vi "ExSpectralCalMovCollect.vi"() -> ()   [LabVIEW 2010]
panel:
  out "XY Graph":T1(graph)
  in  "Pixel Width (microns)":dbl=25.0 format="%.2f"
  in  "Magnification":dbl=1.0 format="%.2f"
  in  "Detector Angle (degrees)":dbl=1.0 format="%.2f"
  in  "Inclusion Angle (degrees)":dbl=1.0 format="%.2f"
  in  "Focal Length (mm)":dbl=300.0 format="%.2f"
  in  "Slope Adjust":dbl format="%.2f"
  in  "Center Offset":dbl format="%.2f"
  out "Current Wavelength":string
  in  "Increment Wavelength":dbl=50.0 format="%.2f"
  in  "End Wavelength":dbl=700.0 format="%.2f"
  in  "Start Wavelength":dbl format="%.2f"
  in  "Grating Speed":dbl=2000.0 min=1.0 step=1.0 format="%.2f"
  in  "Grating number":i16=1 min=1 max=100 step=1
  in  "Temperature":dbl=-10.0 format="%.2f"
  in  "Exposure":dbl min=0.0 step=0.001 format="%.3f"
  in  "stop":bool
  out "error out":errorcluster
  in  "error in (no error)":errorcluster
  # "ExSpectralCalMovCollect.vi\n(Normal Spectrograph via\nUSB/COM port)\nNote that appropriate calibration\ninformation for the spectrometer\nmust be entered before running.Camera and Spectrometer control.  This vi will open both the camera and spectrograph.  It will then move the grating to the Start Wavelength.  Data will then be collected and displayed.  The sequence will be repeated after moving the grating by the Increment Wavelength until the End Wavelength is reached.  At that time, data collection will continue until the STOP button is hit. The display will\nshow an updated calibration in nm."
  # "NOTES:\nIf required, a properly configured camera .ini file must be present for camera operation.\n\nThe properly configured spectrometer .ini file must be present in the LabVIEW folder for spectrograph operation.\n\nConsult the documentation for more information on how to configure these files."
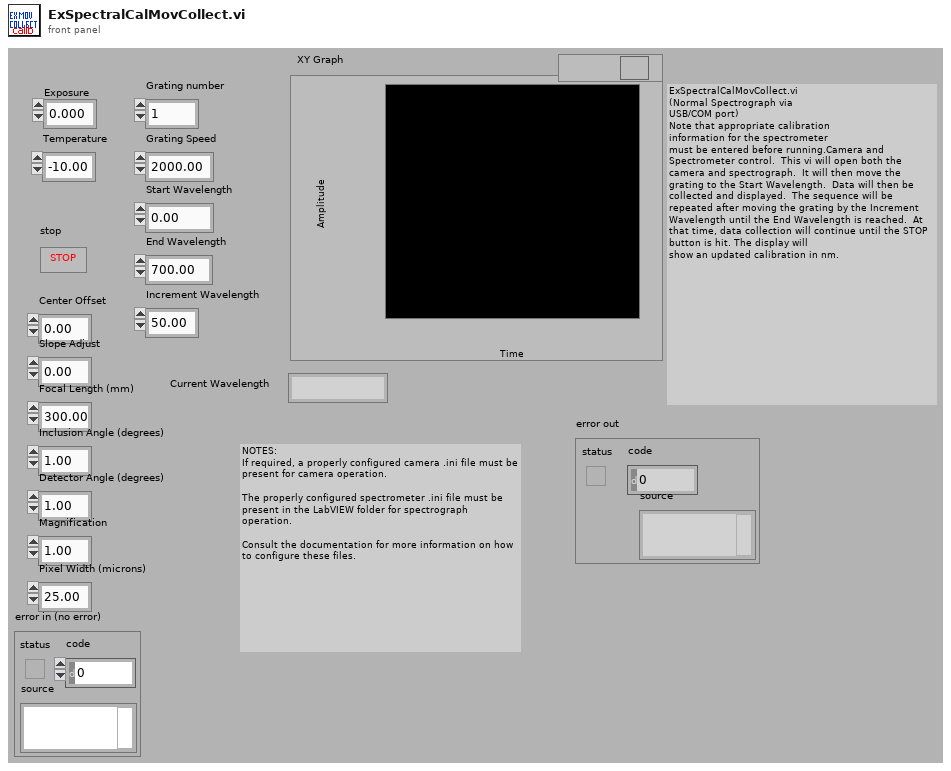
[diagram p1: front panel]
types:
  T1 = cluster{"Calibrated Array":dbl[], "Array F32":sgl[]}
  T2 = cluster{"Center Offset":dbl, "Slope Adjust":dbl, "Focal Length (mm)":dbl, "Inclusion Angle (degrees)":dbl, "Detector Angle (degrees)":dbl, "Magnification":dbl, "Pixel Width (microns)":dbl}
  T3 = cluster{"Camera Handle":u32, "Pulser Handle":u32, "File Handle":u32, "Display Handle":u32, "Image Handle":u32}
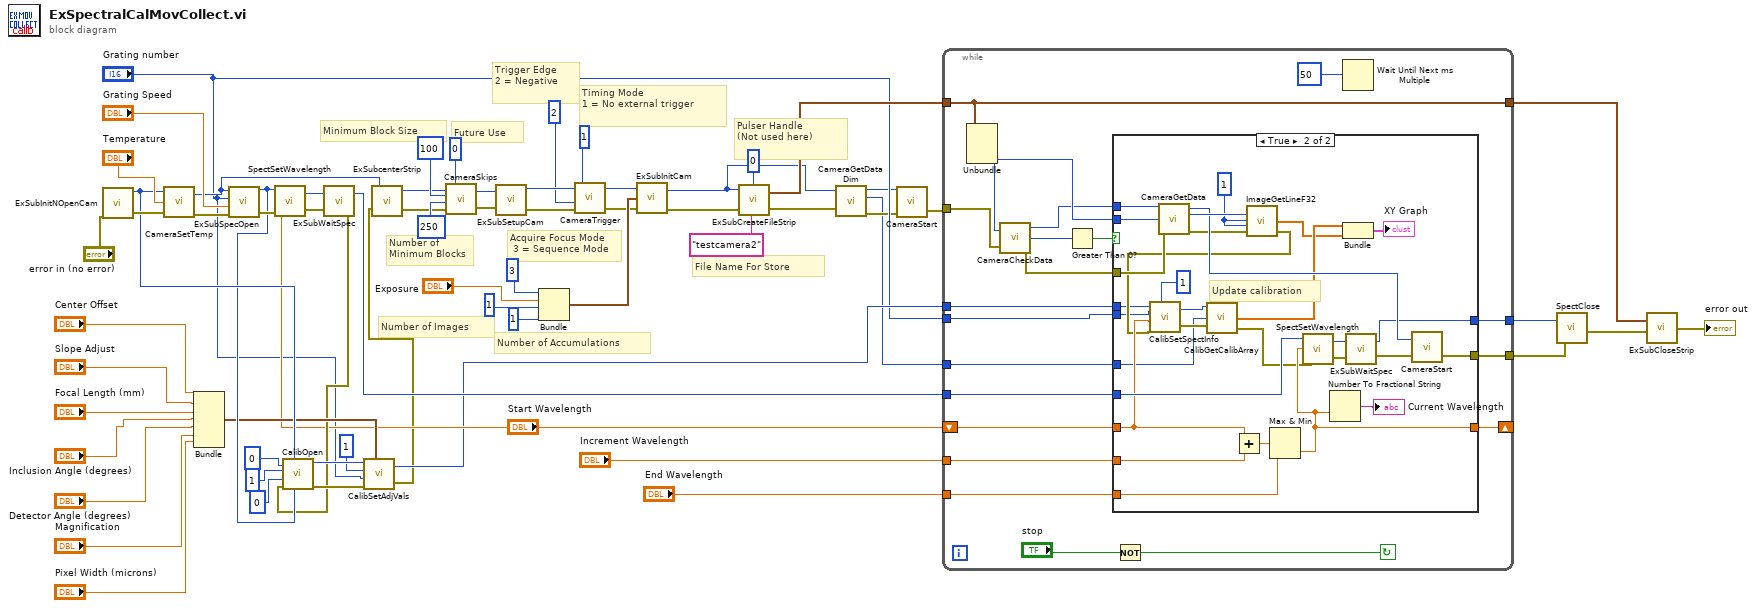
[diagram p0: block diagram]
diagram:
  # "Pulser Handle\n(Not used here)"
  # "Trigger Edge\n2 = Negative"
  # "Timing Mode\n1 = No external trigger"
  # "Future Use"
  # "Number of Minimum Blocks"
  # "Minimum Block Size"
  # "Number of Images"
  # "Number of Accumulations"
  # "Acquire Focus Mode\n 3 = Sequence Mode"
  # "File Name For Store"
  n1 = call "ExSubInitNOpenCam.vi"("error in (no error)"="error in (no error)") -> ("Camera Handle"=w25:u32, "error out"=w29:errorcluster)
  n2 = call <userlib>:"CameraSetTemp.vi"("error in (no error)"=w29, "Temperature"="Temperature", "Camera Handle"=w25) -> ("error out"=w30:errorcluster, "Camera Handle"=w22:u32)
  n3 = Bundle("Center Offset"="Center Offset", "Slope Adjust"="Slope Adjust", "Focal Length (mm)"="Focal Length (mm)", "Inclusion Angle (degrees)"="Inclusion Angle (degrees)", "Detector Angle (degrees)"="Detector Angle (degrees)", "Magnification"="Magnification", "Pixel Width (microns)"="Pixel Width (microns)") -> (w14:T2)  [unwired: 1 in]
  n4 = call "ExSubSpecOpen.vi"("error in (no error)"=w30, "Grating speed"="Grating Speed", "Grating number"="Grating number", "Camera Handles"=w22) -> ("error out"=w35:errorcluster, "Spectrometer Handle"=w23:u32)  [unwired: 1 out]
  n5 = call <userlib>:"SpectSetWavelength.vi"("error in"=w35, "Wavelength"="Start Wavelength", "Spectrometer Handle"=w23) -> ("error out"=w39:errorcluster, "Spectrumeter Handle"=w38:u32)
  n6 = call "ExSubWaitSpec.vi"("error in (no error)"=w39, "Spectrometer Handle"=w38) -> ("error out"=w10:errorcluster, "Spectrometer handle"=w37:u32)
  n7 = call <userlib>:"CalibOpen.vi"("Spectrometer Handle"=w23, "Detector Handle"=w25, "error in"=w10, "Detector Position"=0, "Calibration Type"=1, "Calibration Device ID"=0) -> ("error out"=w12:errorcluster, "Calibration Handle"=w13:u32)
  n8 = call <userlib>:"CalibSetAdjVals.vi"("Calibration Handle"=w13, "Turret Number"=1, "Grating Number"="Grating number", "error in"=w12, "Spectrometer Calibration Parameters"=w14) -> ("Calibration Handle"=w8:u32, "error out"=w6:errorcluster)
  n9 = call "ExSubcenterStrip.vi"("error in (no error)"=w6, "Camera Handle"=w22) -> ("error out"=w41:errorcluster, "Camera Handle"=w42:u32)
  n10 = call <userlib>:"CameraSkips.vi"("Camera Handle"=w42, "Minimum Block Size"=100, "Number of Minimum blocks"=250, "error in"=w41, "Type of Skips"=0) -> ("Camera Handle"=w44:u32, "error out"=w43:errorcluster)
  n11 = call "ExSubSetupCam.vi"("error in (no error)"=w43, "Camera Handle"=w44) -> ("error out"=w49:errorcluster, "Camera Handle"=w53:u32)
  n12 = Bundle(3, "Exposure"="Exposure", 1, 1) -> (w60:cluster{i32, "Exposure":dbl, i32, i32})  [unwired: 1 in]
  n13 = call <userlib>:"CameraTrigger.vi"("error in"=w49, "Trigger Edge"=2, "Timing Mode"=1, "Camera Handle"=w53) -> ("error out"=w54:errorcluster, "Camera Handle"=w52:u32)
  n14 = call "ExSubInitCam.vi"("error in (no error)"=w54, "Camera Information"=w60, "Camera Handle"=w52) -> ("error out"=w59:errorcluster, "Camera Handle"=w5:u32)
  n15 = call "ExSubCreateFileStrip.vi"("error in (no error)"=w59, "File and Display Name"="testcamera2", "Pulser Handle"=0, "Camera Handle"=w5) -> ("error out"=w4:errorcluster, "Handles Out"=w57:T3)
  n16 = call <userlib>:"CameraGetDataDim.vi"("Camera Handle"=w5, "error in"=w4) -> ("Camera Handle"=w2:u32, "Xdim"=w1:u32, "error out"=w3:errorcluster)  [unwired: 1 out]
  n17 = call <userlib>:"CameraStart.vi"("error in"=w3, "Camera Handle"=w2) -> ("error out"=w45:errorcluster)  [unwired: 1 out]
  n18 = while {
    tunnel: w57 -> [w84]
    tunnel: w45 -> [w83]
    tunnel: [w81] -> w31
    tunnel: [w84] -> w56
    tunnel: w37 -> [w75]
    tunnel: "Increment Wavelength" -> [w74]
    tunnel: "End Wavelength" -> [w73]
    shift-right: [w71] -> _
    shift-left: "Start Wavelength" -> [w72]
    tunnel: [w70] -> w32
    tunnel: w8 -> [w69]
    tunnel: "Grating number" -> [w68]
    tunnel: w1 -> [w67]
    stop <- w85 continue-if-true
    n19 = Unbundle(w84) -> ("Camera Handle"=w79:u32, "Image Handle"=w80:u32)  [unwired: 3 out]
    n20 = call <userlib>:"CameraCheckData.vi"("Camera Handle"=w79, "error in"=w83) -> ("Camera Handle"=w78:u32, "Number Of Frames Available"=w76:i32, "error out"=w82:errorcluster)
    n21 = Greater Than 0?(x=w76) -> (x > 0?=w77:bool)
    n22 = case shown="True" w77 {
      tunnel: w82 -> [w90 w120]
      tunnel: [w90 w108] -> w81
      tunnel: w80 -> [_ w117]
      tunnel: w78 -> [_ w116]
      tunnel: w75 -> [w88 w112]
      tunnel: w74 -> [_ w106]
      tunnel: w73 -> [_ w111]
      tunnel: w72 -> [w89 w102]
      tunnel: [w89 w105] -> w71
      tunnel: [w88 w104] -> w70
      tunnel: w69 -> [_ w100]
      tunnel: w68 -> [_ w99]
      tunnel: w67 -> [_ w91]
      frame False {
      }
      frame True {
        w118 = 1
        # "Update calibration"
        n23 = call <userlib>:"CameraGetData.vi"("error in"=w120, "Data Handle"=w117, "Camera Handle"=w116) -> ("error out"=w109:errorcluster, "Data Handle"=w119:u32, "Camera Handle"=w115:u32)
        n24 = Add(x=w102, y=w106) -> (x+y=w110:dbl)
        n25 = call <userlib>:"ImageGetLineF32.vi"("error in"=w109, "Z Position"=w118, "Y Position"=w118, "Data Handle"=w119) -> ("error out"=w101:errorcluster, "Array F32"=w93:sgl[])  [unwired: 1 out]
        n26 = call <userlib>:"CalibSetSpectInfo.vi"("Calibration Handle"=w100, "Current Grating Number"=w99, "Current Wavelength"=w102, "error in"=w101, "Current Turret Number"=1) -> ("Calibration Handle"=w96:u32, "error out"=w97:errorcluster)
        n27 = call <userlib>:"CalibGetCalibArray.vi"("error in"=w97, "Array Size"=w91, "Calibration Handle"=w96) -> ("error out"=w95:errorcluster, "Calibrated Array"=w94:dbl[])  [unwired: 1 out]
        n28 = Max & Min(x=w110, y=w111) -> (min(x,y)=w105:dbl)  [unwired: 1 out]
        n29 = call <userlib>:"SpectSetWavelength.vi"("error in"=w95, "Wavelength"=w105, "Spectrometer Handle"=w112) -> ("error out"=w114:errorcluster, "Spectrumeter Handle"=w113:u32)
        n30 = Number To Fractional String(number=w105) -> (F-format string=→"Current Wavelength":string)  [unwired: 3 in]
        n31 = Bundle("Calibrated Array"=w94, "Array F32"=w93) -> (→"XY Graph":T1)  [unwired: 1 in]
        n32 = call "ExSubWaitSpec.vi"("error in (no error)"=w114, "Spectrometer Handle"=w113) -> ("error out"=w103:errorcluster, "Spectrometer handle"=w104:u32)
        n33 = call <userlib>:"CameraStart.vi"("error in"=w103, "Camera Handle"=w115) -> ("error out"=w108:errorcluster)  [unwired: 1 out]
      }
    }
    n34 = Not(x="stop") -> (.not. x?=w85:bool)
    n35 = Wait Until Next ms Multiple(millisecond multiple=50) -> ()  [unwired: 1 out]
  }
  n36 = call <userlib>:"SpectClose.vi"("error in"=w31, "Spectrometer Handle"=w32) -> ("error out"=w33:errorcluster)
  n37 = call "ExSubCloseStrip.vi"("error in (no error)"=w33, "Handles In"=w56) -> ("error out"=→"error out":errorcluster)
